vi "JL_EnterServiceMode.vi"(0 "GEA2 Reference In":refnum<k24>, 1 "Erd_KeyStatusWordSelector ERD #":T1={"ERD Number"=61536, "Data Type"=enum."string", "Data"=""} {"ERD Number" format="%.0x"}, 2 "Erd_KnobSelector ERD #":T1={"ERD Number"=61532, "Data Type"=enum."string", "Data"=""} {"ERD Number" format="%.0x"}, 5 "MC GEA Inputs":T3={"Source"=228, "Destination"=36} {"Destination" format="%.0x"; "Source" format="%.0x"}, 7 "UI GEA Inputs":T3={"Source"=228, "Destination"=37} {"Destination" format="%.0x"; "Source" format="%.0x"}, 9 "Hold Time (s)":dbl=7.0 format="%#_13g", 11 "Error In":errorcluster, 12 "Erd_AutomationKeyStatusWord ERD #":T1={"ERD Number"=61535, "Data Type"=enum."string", "Data"=""} {"ERD Number" format="%.0x"}, 13 "Erd_KnobAutomationData ERD #":T1={"ERD Number"=61534, "Data Type"=enum."string", "Data"=""} {"ERD Number" format="%.0x"}) -> (4 "GEA2 Reference Out":refnum<k24>, 15 "Error Out":errorcluster)   [LabVIEW 2016]
uses:
  Q:/Common/DLLs/GEA3/GeaCommunication.dll
  Common/DLLs/GEA3/GeaCommunication.dll
  Common/LabVIEW GEA2 Toolkit/LabVIEW_GEA2_Toolkit.lvlibp/type defs/Source_Destination.ctl
  Common/LabVIEW GEA2 Toolkit/LabVIEW_GEA2_Toolkit.lvlibp/type defs/ERD Write Data In.ctl
  Common/LabVIEW GEA2 Toolkit/LabVIEW_GEA2_Toolkit.lvlibp/type defs/Data Type.ctl
  Common/LabVIEW GEA2 Toolkit/LabVIEW_GEA2_Toolkit.lvlibp/type defs/ERD Read Data In.ctl
  <vilib>/DAQmx/write.llb/DAQmx Write (Digital Bool 1Line 1Point).vi
  <vilib>/DAQmx/create/channels.llb/DAQmx Create Channel (DO-Digital Output).vi
  <vilib>/DAQmx/miscellaneous.llb/DAQmx Fill In Error Info.vi
  Common/LabVIEW GEA2 Toolkit/LabVIEW_GEA2_Toolkit.lvlibp
panel:
  in  "Model":enum16{"Estar Centauro", "TL27SB"}(ring)
  in  "SLB?":bool=TRUE
  in  "Board Index":i32
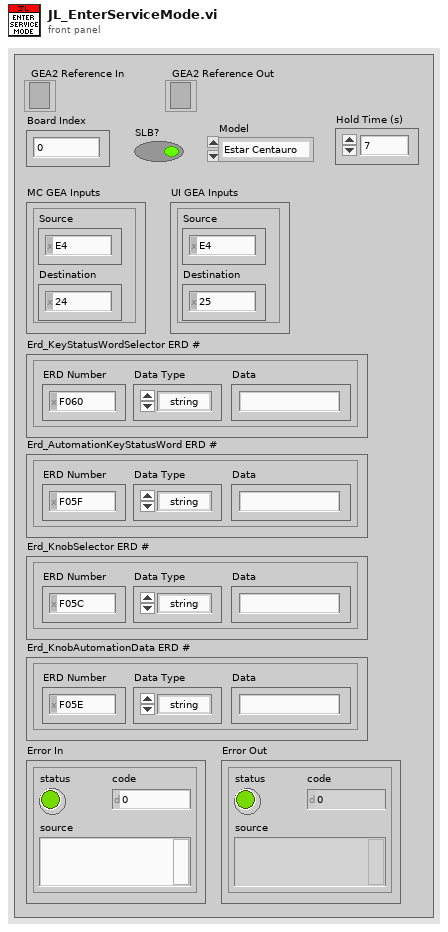
[diagram p1: front panel]
types:
  T1 = typedef "LabVIEW_GEA2_Toolkit.lvlibp/ERD Write Data In.ctl" = cluster{"ERD Number":u16, "Data Type":T2, "Data":string}
  T2 = typedef "LabVIEW_GEA2_Toolkit.lvlibp/Data Type.ctl" = enum16{"string", "boolean", "uint8_t", "uint16_t", "uint32_t", "uint64_t", "int8_t", "int16_t", "int32_t", "int64_t"}
  T3 = typedef "LabVIEW_GEA2_Toolkit.lvlibp/Source_Destination.ctl" = cluster{"Source":u8, "Destination":u8}
  T4 = typedef "LabVIEW_GEA2_Toolkit.lvlibp/ERD Read Data In.ctl" = cluster{"ERD Number":u16, "Data Type":T2}
  T5 = typedef "LabVIEW_GEA2_Toolkit.lvlibp/ERD Read Data Out.ctl" = cluster{"ERD Number":u16, "Data":string}
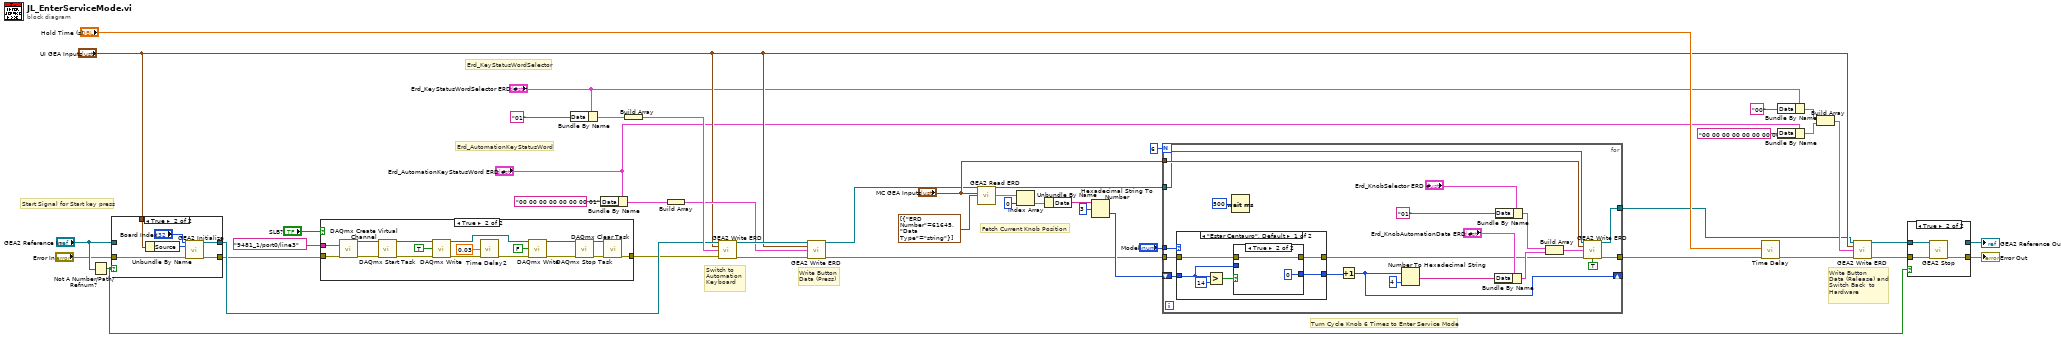
[diagram p0: block diagram]
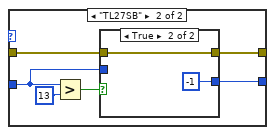
[diagram p3: hidden frame]
diagram:
  # "Erd_AutomationKeyStatusWord"
  # "Erd_KeyStatusWordSelector"
  # "Fetch Current Knob Position"
  # "Turn Cycle Knob 6 Times to Enter Service Mode"
  # "Start Signal for Start key press"
  # "Write Button\nData (Release) and \nSwitch Back  to\nHardware"
  # "Write Button\nData (Press)"
  # "Switch to\nAutomation \nKeyboard"
  n1 = Not A Number/Path/Refnum?(number/path/refnum="GEA2 Reference In") -> (NaN/Path/Refnum?=w42:bool)
  n2 = case shown="True" w42 {
    tunnel: "Error In" -> [w46 w53]
    tunnel: [w46 w52] -> w25
    tunnel: "GEA2 Reference In" -> [w47 _]
    tunnel: [w47 w51] -> w30
    tunnel: "UI GEA Inputs" -> [_ w49]
    frame False {
    }
    frame True {
      n3 = Unbundle By Name(w49) -> ("Source"=w50:u8)
      n4 = call "GEA2 Initialize.vi"("Board Index"="Board Index", "Source Address"=w50, "error in"=w53) -> ("GEA2 Reference Out"=w51:refnum<k24>, "error out"=w52:errorcluster)  [unwired: 10 in, 1 out]
    }
  }
  n5 = case shown="True" "SLB?" {
    tunnel: tag "9481_1/port0/line3" ("Line(s)") -> [_ w65]
    tunnel: [w54 w62] -> w24
    tunnel: w25 -> [w54 w58]
    frame False {
    }
    frame True {
      n6 = call-poly <vilib>:"DAQmx Create Virtual Channel.vi"("lines"=w65, "error in"=w58) -> ("task out"=w68:refnum<k21>, "error out"=w69:errorcluster)  [unwired: 12 in]
      n7 = call <vilib>:"DAQmx Start Task.vi"("task/channels in"=w68, "error in"=w69) -> ("task out"=w71:refnum<k21>, "error out"=w70:errorcluster)  [unwired: 12 in]
      n8 = call-poly <vilib>:"DAQmx Write.vi"("task/channels in"=w71, "data"=TRUE ("Boolean"), "error in"=w70) -> ("task out"=w59:refnum<k21>, "error out"=w61:errorcluster)  [unwired: 10 in, 1 out]
      n9 = call "Time Delay2"("error in (no error)"=w61, "Delay Time (s)"=0.03) -> ("error out"=w60:errorcluster)  [unwired: 9 in]
      n10 = call-poly <vilib>:"DAQmx Write.vi"("task/channels in"=w59, "data"=FALSE ("Boolean"), "error in"=w60) -> ("task out"=w64:refnum<k21>, "error out"=w63:errorcluster)  [unwired: 10 in, 1 out]
      n11 = call <vilib>:"DAQmx Stop Task.vi"("task/channels in"=w64, "error in"=w63) -> ("task out"=w67:refnum<k21>, "error out"=w66:errorcluster)  [unwired: 12 in]
      n12 = call <vilib>:"DAQmx Clear Task.vi"("task in"=w67, "error in"=w66) -> ("error out"=w62:errorcluster)  [unwired: 13 in]
    }
  }
  n13 = Bundle By Name(cluster="Erd_KeyStatusWordSelector ERD #", "Data"="01") -> (w41:T1)
  n14 = Bundle By Name(cluster="Erd_AutomationKeyStatusWord ERD #", "Data"="00 00 00 00 00 00 00 01") -> (w5:T1)
  n15 = Build Array(w41) -> (w40:T1[])
  n16 = Build Array(w5) -> (w33:T1[])
  n17 = call "GEA2 Write ERD.vi"("GEA2 Reference In"=w30, "GEA Inputs"="UI GEA Inputs", "Write ERD List"=w40, "Error In"=w24) -> ("GEA2 Reference Out"=w34:refnum<k24>, "Error Out"=w35:errorcluster)  [unwired: 9 in, 1 out]
  n18 = call "GEA2 Write ERD.vi"("GEA2 Reference In"=w34, "GEA Inputs"="UI GEA Inputs", "Write ERD List"=w33, "Error In"=w35) -> ("GEA2 Reference Out"=w13:refnum<k24>, "Error Out"=w9:errorcluster)  [unwired: 9 in, 1 out]
  n19 = call "GEA2 Read ERD.vi"("GEA2 Reference In"=w13, "GEA Inputs"="MC GEA Inputs", "Read ERD List"=T4[] [{"ERD Number"=61645, "Data Type"=enum."string"}]) -> ("GEA2 Reference Out"=w12:refnum<k24>, "ERD Data Out"=w21:T5[])  [unwired: 9 in, 2 out]
  n20 = Index Array(array=w21, index=0) -> (element=w19:T5)
  n21 = Unbundle By Name(w19) -> ("Data"=w18:string)
  n22 = Hexadecimal String To Number(string=w18, offset=3) -> (number=w16:u32)  [unwired: 1 in, 1 out]
  n23 = for {
    N: 6 -> [_]
    tunnel: "MC GEA Inputs" -> [w83]
    shift-right: [w78] -> _
    shift-left: w16 -> [w82]
    tunnel: "Model" -> [w80]
    tunnel: w12 -> [w77]
    tunnel: [w76] -> w11
    tunnel: [w75] -> w10
    tunnel: w9 -> [w74]
    n24 = case shown="\"Estar Centauro\", Default" w80 {
      tunnel: w82 -> [w96 w105]
      tunnel: [w95 w104] -> w79
      tunnel: w74 -> [w93 w103]
      tunnel: [w94 w102] -> w73
      frame "Estar Centauro", Default {
        n25 = Greater?(x=w96, y=u32 14) -> (0:w97:bool)
        n26 = case shown="True" w97 {
          tunnel: w96 -> [w99 _]
          tunnel: [w99 0] -> w95
          tunnel: [w98 w100] -> w94
          tunnel: w93 -> [w98 w100]
          frame False {
          }
          frame True {
          }
        }
      }
      frame "TL27SB" {
        n27 = Greater?(x=w105, y=u32 13) -> (0:w106:bool)
        n28 = case shown="True" w106 {
          tunnel: w105 -> [w109 _]
          tunnel: [w109 -1] -> w104
          tunnel: w103 -> [w108 w110]
          tunnel: [w108 w110] -> w102
          frame False {
          }
          frame True {
          }
        }
      }
    }
    n29 = Wait (ms)(milliseconds to wait=u32 500) -> ()  [unwired: 1 out]
    n30 = Increment(x=w79) -> (x+1=w78:u32)
    n31 = Number To Hexadecimal String(1:i16 4 ("width (-)"), 2:w78) -> (0:w90:string)
    n32 = Bundle By Name(cluster="Erd_KnobAutomationData ERD #", "Data"=w90) -> (w86:T1)
    n33 = Bundle By Name(cluster="Erd_KnobSelector ERD #", "Data"="01" ("Message")) -> (w87:T1)
    n34 = Build Array(w87, w86) -> (w85:T1[])
    n35 = call "GEA2 Write ERD.vi"("GEA2 Reference In"=w77, "GEA Inputs"=w83, "Write ERD List"=w85, "Error In"=w73, "Verify ERD Response?"=TRUE) -> ("GEA2 Reference Out"=w76:refnum<k24>, "Error Out"=w75:errorcluster)  [unwired: 8 in, 1 out]
  }
  n36 = call "Time Delay"("error in (no error)"=w10, "Delay Time (s)"="Hold Time (s)") -> ("error out"=w38:errorcluster)  [unwired: 9 in]
  n37 = Bundle By Name(cluster="Erd_KeyStatusWordSelector ERD #", "Data"="00") -> (w1:T1)
  n38 = Bundle By Name(cluster="Erd_AutomationKeyStatusWord ERD #", "Data"="00 00 00 00 00 00 00 00") -> (w2:T1)
  n39 = Build Array(w1, w2) -> (w39:T1[])
  n40 = call "GEA2 Write ERD.vi"("GEA2 Reference In"=w11, "GEA Inputs"="UI GEA Inputs", "Write ERD List"=w39, "Error In"=w38) -> ("GEA2 Reference Out"=w36:refnum<k24>, "Error Out"=w37:errorcluster)  [unwired: 9 in, 1 out]
  n41 = case shown="True" w42 {
    tunnel: [w112 w116] -> w45
    tunnel: w36 -> [w113 w115]
    tunnel: [w113 _] -> w44
    tunnel: w37 -> [w112 w114]
    frame False {
    }
    frame True {
      n42 = call "GEA2 Stop.vi"("GEA2 Reference In"=w115, "Error In"=w114) -> ("Error Out"=w116:errorcluster)  [unwired: 13 in]
    }
  }
  "Error Out" <- w45
  "GEA2 Reference Out" <- w44
